vi "Write ini.vi"(9 "configuration file path":path=path "C:/Users/hzy/Desktop/配置.ini" caption="配置文件的路径", 10 "数组":string[][](array[string]), 11 "段":string) -> ()   [LabVIEW 2021]
uses:
  <vilib>/Utility/config.llb/Write Key (String).vi
  <vilib>/Utility/config.llb/NI_LVConfig.lvlib
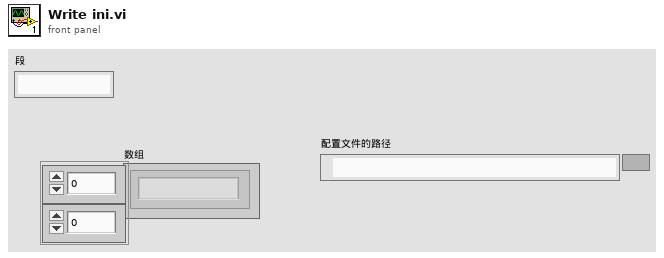
[diagram p1: front panel]
types:
  T1 = typedef "NI_LVConfig.lvlib/Config Data RefNum.ctl" = refnum<k1>
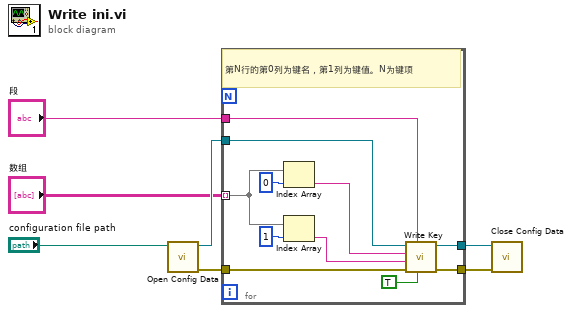
[diagram p0: block diagram]
diagram:
  n1 = call <vilib>:"Open Config Data.vi"("configuration file path"="configuration file path") -> ("error out"=w5:errorcluster, "refnum"=w6:T1)  [unwired: 8 in, 1 out]
  n2 = for {
    tunnel: "数组" -> [w12] mode=indexing
    tunnel: w6 -> [w18]
    tunnel: [w15] -> w3
    tunnel: w5 -> [w17]
    tunnel: [w16] -> w4
    tunnel: "段" -> [w9]
    # "第N行的第0列为键名，第1列为键值。N为键项"
    n3 = Index Array(array=w12, index=0 ("索引")) -> (element=w13:string)
    n4 = Index Array(array=w12, index=1 ("索引")) -> (element=w10:string)
    n5 = call-poly <vilib>:"Write Key.vi"("write raw string? (F)"=TRUE, "section"=w9, "error in (no error)"=w17, "value"=w10, "key"=w13, "refnum"=w18) -> ("error out"=w16:errorcluster, "refnum out"=w15:T1)  [unwired: 3 in, 1 out]
  }
  n6 = call <vilib>:"Close Config Data.vi"("error in (no error)"=w4, "refnum"=w3) -> ()  [unwired: 8 in, 2 out]
